vi "testclient.vi"() -> ()   [LabVIEW 2016]
uses:
  tls classes/engine context/engine context.lvclass
  tls classes/connection creator/client connector/client connector.lvclass
  tls classes/connection/connection.lvclass
panel:
  out "error out":errorcluster
  out "Array":cluster{"error code":i32, "data":string}[](array[cluster])
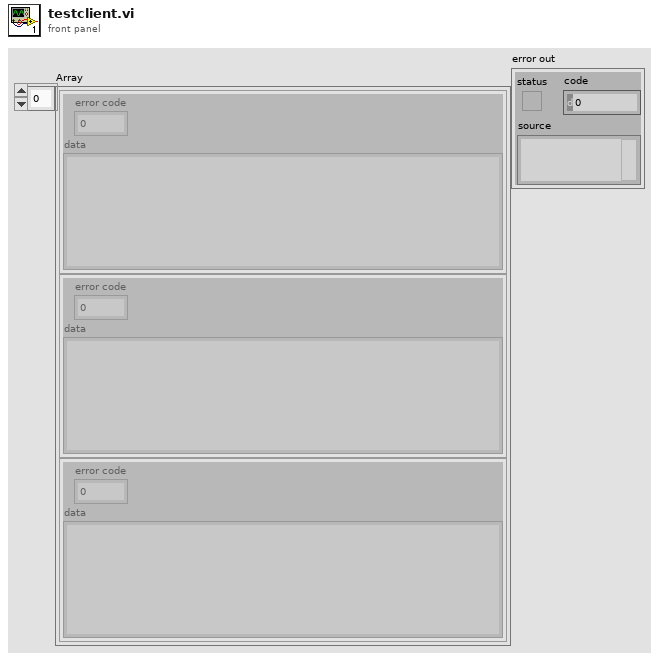
[diagram p1: front panel]
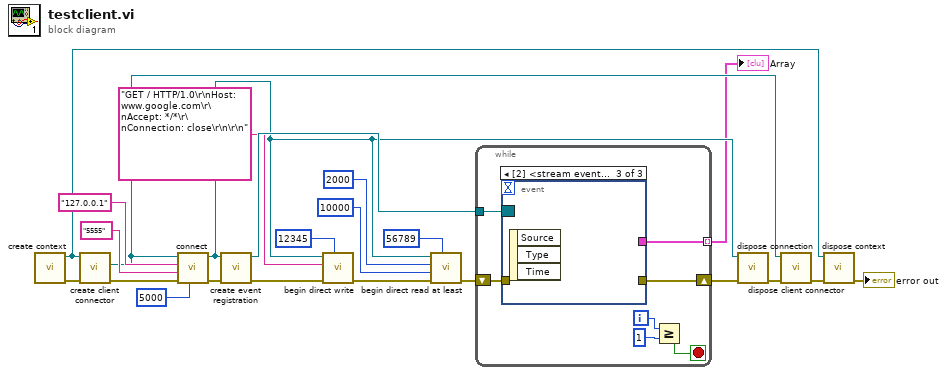
[diagram p0: block diagram]
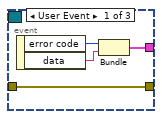
[diagram p2: hidden frame]
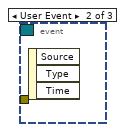
[diagram p3: hidden frame]
diagram:
  n1 = call "create context.vi"() -> ("error out"=w23:errorcluster, "engine context out"=w4:refnum<class "engine context.lvclass">)  [unwired: 10 in]
  n2 = call "create client connector.vi"("error in"=w23, "engine context in"=w4) -> ("error out"=w22:errorcluster, "client connector out"=w6:refnum<class "client connector.lvclass">)  [unwired: 8 in]
  n3 = call "connect.vi"("timeout"=5000, "error in"=w22, "port"="5555", "host"="127.0.0.1", "client connector in"=w6) -> ("error out"=w18:errorcluster, "connection out"=w8:refnum<class "connection.lvclass">)  [unwired: 5 in]
  n4 = call "create event registration.vi"("error in"=w18, "connection in"=w8) -> ("error out"=w15:errorcluster, "Event Registration Refnum"=w17:refnum<event-registration>)  [unwired: 8 in]
  n5 = call "begin direct write.vi"("id"=u32 12345, "error in"=w15, "data"="GET / HTTP/1.0\r\nHost: www.google.com\r\nAccept: */*\r\nConnection: close\r\n\r\n", "connection in"=w8) -> ("error out"=w13:errorcluster)  [unwired: 7 in]
  n6 = call "begin direct read at least.vi"("id"=u32 56789, "error in"=w13, "max bytes to read"=10000 ("bytes to read"), "min bytes to read"=2000 ("bytes to read"), "connection in"=w8) -> ("error out"=w9:errorcluster)  [unwired: 6 in]
  n7 = while {
    tunnel: w17 -> [w30]
    tunnel: [w28] -> w3 mode=indexing
    shift-right: [w24] -> w2
    shift-left: w9 -> [w29]
    i -> [w27]
    stop <- w25 stop-if-true
    n8 = event shown="[2] <stream event>: User Event" {
      selector: w30 -> [_ _ _]
      dyn-events: _ -> [_ _ _]
      timeout: _ -> [_ _ _]
      tunnel: w29 -> [w31 _ _]
      tunnel: [w32 _ _] -> w28
      tunnel: [w31 _ _] -> w24
      event User Event {
        n9 = event-data() -> ("error code"=w33:i32, "data"=w34:string)  [unwired: 1 in]
        n10 = Bundle("error code"=w33, "data"=w34) -> (w32:cluster{"error code":i32, "data":string})  [unwired: 1 in]
      }
      event User Event {
        n11 = event-data() -> ()  [unwired: 1 in, 3 out]
      }
      event User Event {
        n12 = event-data() -> ()  [unwired: 1 in, 3 out]
      }
    }
    n13 = Greater Or Equal?(x=w27, y=1) -> (x >= y?=w25:bool)
  }
  "Array" <- w3
  n14 = call "dispose connection.vi"("error in"=w2, "connection in"=w8) -> ("error out"=w7:errorcluster)  [unwired: 9 in]
  n15 = call "dispose client connector.vi"("error in"=w7, "client connector in"=w6) -> ("error out"=w5:errorcluster)  [unwired: 9 in]
  n16 = call "dispose context.vi"("error in"=w5, "engine context out"=w4) -> ("error out"=→"error out":errorcluster)  [unwired: 9 in]
